vi "Save Animated GIF Example.vi"() -> ()   [LabVIEW 2020]
doc: "G-Image example demonstrating generating and saving an animation in GIF format."
uses:
  <vilib>/picture/picture.llb/imagedata.ctl
  Image IO/Polymorphic VIs/Save Animated GIF Image (Path).vi
  G-Image.lvlib
panel:
  out "State":string
  out "Waveform Chart":cluster{dbl, dbl}(graph)={-0.06975647374412564, 0.4806308479691592}
  # "Instructions:\n1. Run the VI.\n2. Select a location to save the image file.\n3. A short animation will be created and saved to the file.\n4. Open the image in an image viewer or browser  to view the animation."
  # "G"
  # "-Image"
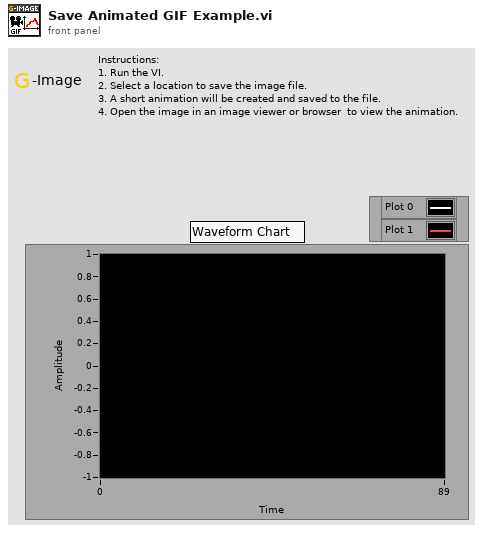
[diagram p1: front panel]
types:
  T1 = typedef "imagedata.ctl" = cluster{"image type":i32, "image depth":i32, "image":u8[], "mask":u8[], "colors":u32[], "Rectangle":cluster{"left":i16, "top":i16, "right":i16, "bottom":i16}}
  T2 = enum16{"File Selection", "Image Generation", "Saving", "Complete"}
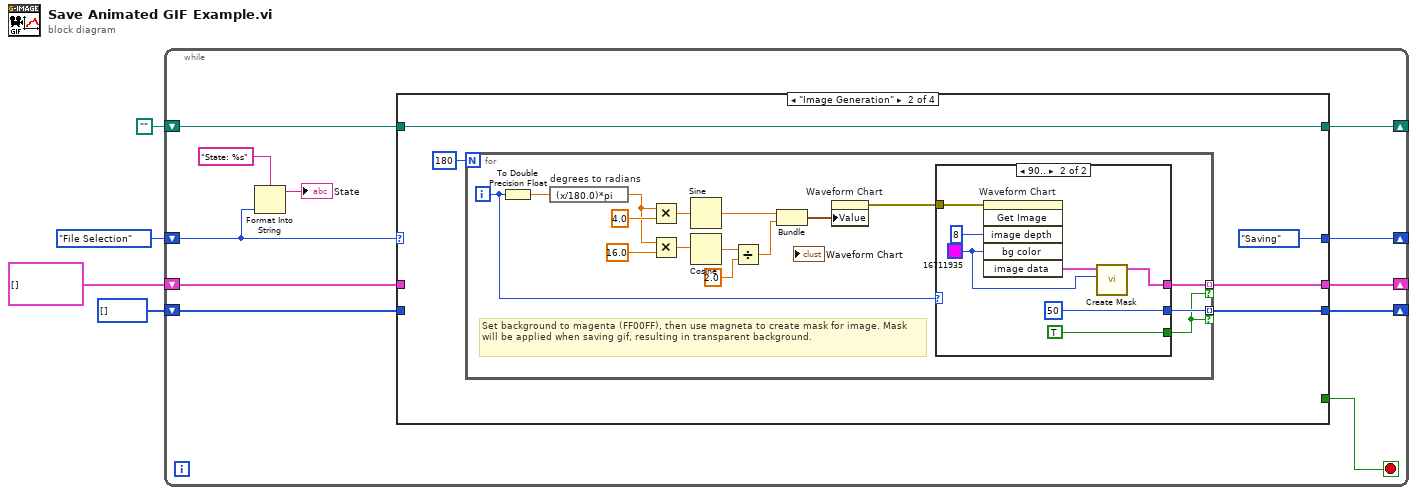
[diagram p0: block diagram]
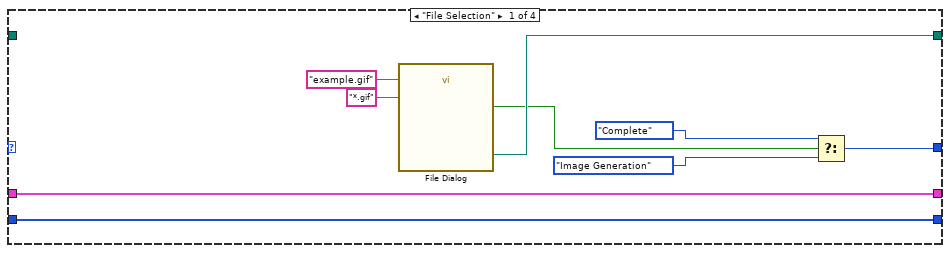
[diagram p2: hidden frame]
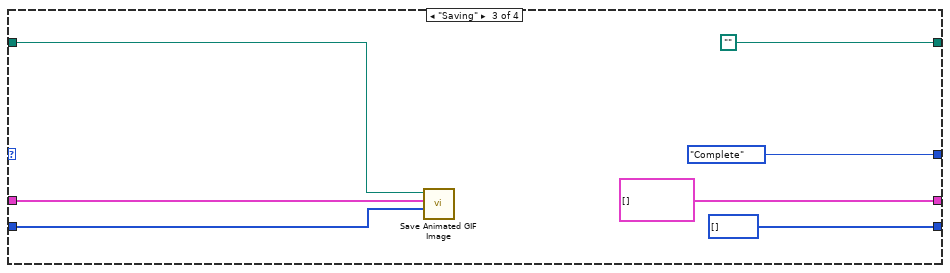
[diagram p4: hidden frame]
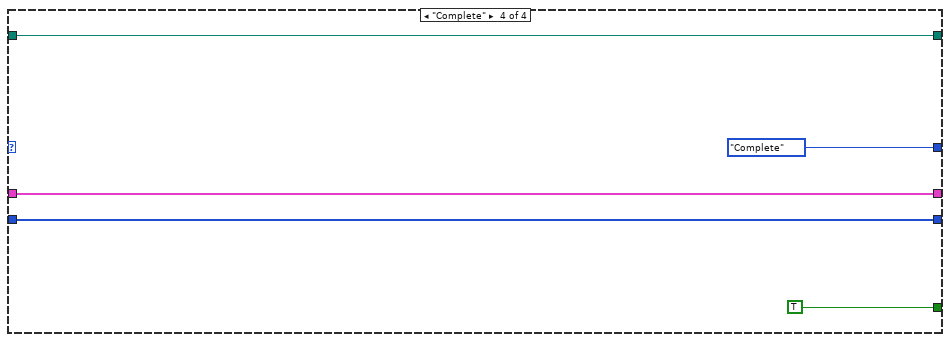
[diagram p5: hidden frame]
diagram:
  n1 = while {
    shift-right: [w5] -> _
    shift-left: T2."File Selection" -> [w9]
    shift-right: [w15] -> _
    shift-left: path "" -> [w14]
    shift-right: [w13] -> _
    shift-left: T1[] [] -> [w11]
    shift-right: [w12] -> _
    shift-left: i32[] [] -> [w10]
    stop <- w6 stop-if-true
    n2 = Format Into String(format string="State: %s", w9) -> (resulting string=→"State":string)  [unwired: 2 in, 1 out]
    n3 = case shown="\"Image Generation\"" w9 {
      tunnel: [w22 w26 path "" w60] -> w15
      tunnel: w14 -> [_ w26 w59 w60]
      tunnel: [w21 w28 T1[] [] w62] -> w13
      tunnel: [w20 w27 i32[] [] w61] -> w12
      tunnel: w11 -> [w21 _ w58 w62]
      tunnel: w10 -> [w20 _ w57 w61]
      tunnel: [_ _ _ TRUE] -> w6
      tunnel: [w16 T2."Saving" T2."Complete" ("f") T2."Complete" ("f")] -> w5
      frame "File Selection" {
        n4 = call "File Dialog"("default name"="example.gif", "pattern (all files)"="*.gif") -> ("selected path"=w22:path, "cancelled"=w19:bool)  [unwired: 10 in, 2 out]
        n5 = Select(t=T2."Complete", s=w19, f=T2."Image Generation") -> (s? t:f=w16:T2)
      }
      frame "Image Generation" {
        n6 = for {
          N: 180 -> [_]
          tunnel: [w45] -> w28 mode=indexing if=w30
          tunnel: [w32] -> w27 mode=indexing if=w30
          i -> [w31]
          # "Set background to magenta (FF00FF), then use magneta to create mask for image. Mask will be applied when saving gif, resulting in transparent background."
          n7 = To Double Precision Float(number=w31) -> (double precision float=w42:dbl)
          n8 = expression code="(x/180.0)*pi" "degrees to radians"(w42) -> (w37:dbl)
          n9 = Multiply(x=w37, y=4.0) -> (x*y=w40:dbl)
          n10 = Multiply(x=w37, y=16.0) -> (x*y=w35:dbl)
          n11 = Sine(x=w40) -> (sin(x)=w39:dbl)
          n12 = Cosine(x=w35) -> (cos(x)=w38:dbl)
          n13 = Divide(x=w38, y=2.0) -> (x/y=w34:dbl)
          n14 = Bundle(w39, w34) -> (w41:cluster{dbl, dbl})  [unwired: 1 in]
          n15 = property on="Waveform Chart" class="WFChart (strict)"("Value"=w41) -> (error out=w44:errorcluster)  [unwired: 2 in, 1 out]
          n16 = case shown="90.." w31 {
            tunnel: [_ w47] -> w45
            tunnel: w44 -> [_ w51]
            tunnel: [_ 50] -> w32
            tunnel: [_ TRUE] -> w30
            frame Default {
            }
            frame 90.. {
              w46 = u32 16711935 ("Background Color")
              n17 = invoke on="Waveform Chart" class="WFChart (strict)" method="Get Image"(error in=w51, "image depth"=8 ("Image Depth"), "bg color"=w46) -> ("image data"=w48:T1)  [unwired: 3 in, 5 out]
              n18 = call <vilib>:"Create Mask.vi"("Mask Color (Black)"=w46, "image data"=w48) -> ("image data"=w47:T1)  [unwired: 9 in]
            }
          }
        }
      }
      frame "Saving" {
        n19 = call-poly "Save Animated GIF Image.vi"("Delays"=w57, "Frames"=w58, "Path In"=w59) -> ()  [unwired: 7 in, 2 out]
      }
      frame "Complete" {
      }
    }
  }
